vi "Subvi AO.vi"(2 "AO channel":refnum<k21>="Connector1/AO0", 8 "Ext trig enable":bool, 10 "Memory label":refnum<k21>="AO0 buffer") -> ()   [LabVIEW 2017]
uses:
  <vilib>/Platform/TimedLoop/XDataNode/timing_clust.ctl
  <vilib>/Platform/TimedLoop/XDataNode/nitl_modes.ctl
  <vilib>/Platform/TimedLoop/XDataNode/wakeup.ctl
  <vilib>/rvi/Emulation/niFpgaSctlEmulationGetInTimedLoop.vi
  <vilib>/rvi/Emulation/niFpgaEmulationReportErrorSimple.vi
  <vilib>/rvi/Emulation/niFpgaGetClockAttributes.vi
  <vilib>/rvi/Emulation/niFpgaCriticalErrorInLSC.vi
  Detector/GV line clock start.vi
  <vilib>/rvi/DataTransferAndStorage/Container/Common/niFpgaContainerExecOnDevCompGetState.vi
  <vilib>/rvi/Emulation/niFpgaEmulationIsFPGAContextNoSignature.vi
  <vilib>/rvi/DataTransferAndStorage/Container/Common/niFpgaContainerGetUniqueNameForEmu.vi
  <vilib>/rvi/Emulation/niFpgaProcessEmulError.vi
  <vilib>/rvi/errors/nirviReportUnexpectedCaseInternalError (U32).vi
  <vilib>/rvi/Memory/Memory_Emulation/niFpgaMemoryEmulationCacheClearOnFirstRun.vi
  <vilib>/rvi/Memory/Memory_Emulation/nirvimemoryEmulationManagerCache_MakeExclusive.vi
  <vilib>/rvi/Memory/Memory_Emulation/niFpgaMemoryEmulationValidateCache.vi
  <vilib>/rvi/Memory/Memory_Emulation/nirvimemoryEmulationManagerCache_InsertValue.vi
  <vilib>/Utility/error.llb/Clear Errors.vi
  <vilib>/rvi/Memory/Memory_Emulation/nirvimemoryEmulationManagerCache_ReleaseExclusive.vi
  <vilib>/rvi/Memory/Memory_Emulation/nirvimemoryEmulationManagerCache_GetValue.vi
  <vilib>/rvi/Memory/Memory_Emulation/nirvimemoryEmulationManagerCache_SetValue.vi
  <vilib>/rvi/Emulation/niFpgaSctlEmulationResourceMgr.vi
  <vilib>/rvi/eio/common/nirviEmuTemplateMethod_errors.vi
  <vilib>/Platform/TimedLoop/XDataNode/XDataNode.xnode
  <vilib>/rvi/DataTransferAndStorage/Container/XNode/niFpgaContainer.xnode
  <vilib>/rvi/Memory/Memory_Emulation/niFpgaMemoryEmulationRefIn.vi
  <vilib>/eio/EIONode/EIONode.xnode
  <vilib>/Platform/TimedLoop/XDataNode/XDNodeRunTimeDep.lvlib
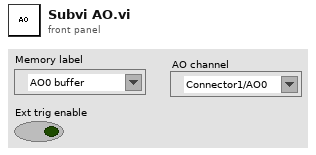
[diagram p1: front panel]
types:
  T1 = typedef "XDNodeRunTimeDep.lvlib/timing_clust.ctl" = cluster{"Expected End [f-1]":u64, "Actual End [f-1]":u64, "Finished Late? [f-1]":bool, "Expected End [i-1]":u64, "Actual End [i-1]":u64, "Finished Late? [i-1]":bool, "Expected Start [i]":u64, "Actual Start [i]":u64, "Expected Start [f]":u64, "Actual Start [f]":u64, "Source Name":string, "Structure Name":string, "Period":i64, "Deadline":i64, "Offset":i64, "Start":i64, "Priority":i32, "Timeout":i32, "Mode":T2, "Wakeup Reason":T3, "Error":errorcluster, "Source Type":string, "Secondary Source Type":string, "Global End Time":u64, "Global Start Time":u64, "Frame Duration":u64, "Iteration Duration":u64, "Assigned CPU":i32, "I/O Scan Engine Mode":u32}
  T2 = typedef "XDNodeRunTimeDep.lvlib/nitl_modes.ctl" = enum32{"No Change", "Process missed periods, maintain original phase", "Discard missed periods, maintain original phase", "Process missed periods, ignore original phase", "Discard missed periods, ignore original phase"}
  T3 = typedef "XDNodeRunTimeDep.lvlib/wakeup.ctl" = enum32{"Normal", "Aborted", "Asynchronous wakeup", "Timing source error", "Timed loop error", "Timeout"}
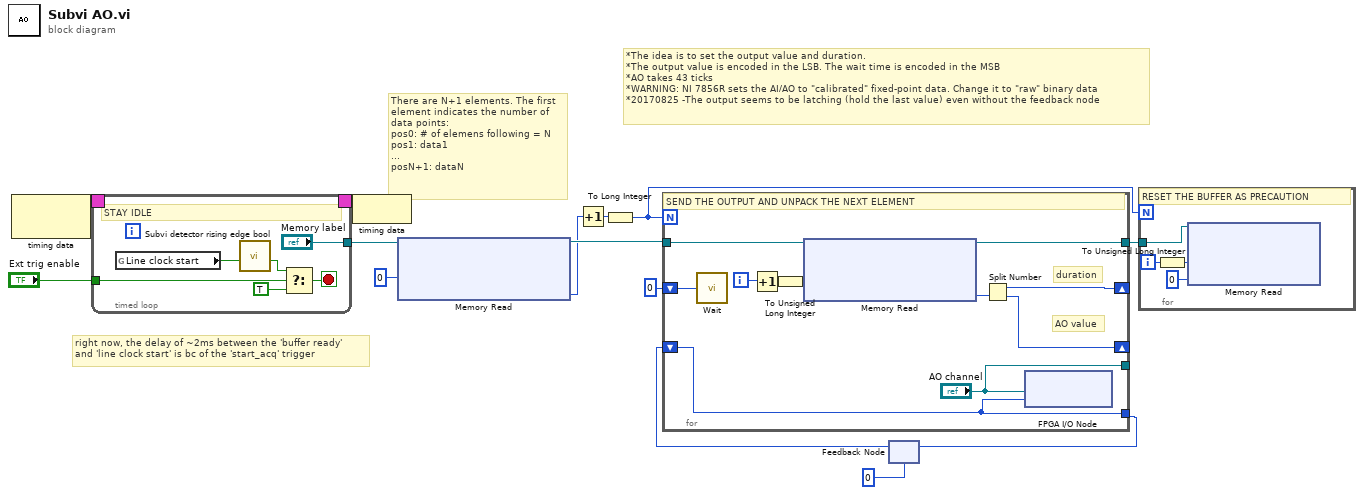
[diagram p0: block diagram]
diagram:
  # "right now, the delay of ~2ms between the 'buffer ready'\nand 'line clock start' is bc of the 'start_acq' trigger"
  # "There are N+1 elements. The first\nelement indicates the number of\ndata points:\npos0: # of elemens following = N\npos1: data1\n...\nposN+1: dataN"
  # "*The idea is to set the output value and duration.\n*The output value is encoded in the LSB. The wait time is encoded in the MSB\n*AO takes 43 ticks\n*WARNING: NI 7856R sets the AI/AO to \"calibrated\" fixed-point data. Change it to \"raw\" binary data\n*20170825 -The output seems to be latching (hold the last value) even without the feedback node"
  n1 = node-c288() -> (w3:T1)  [unwired: 1 in]
  n2 = timed-loop {
    tunnel: ["Memory label"] -> w4
    timing: w3 -> [_]
    timing-out: [_] -> w2
    tunnel: "Ext trig enable" -> [w18]
    stop <- w16 stop-if-true
    # "STAY IDLE"
    n3 = global read "GV line clock start.vi" "Line clock start"() -> (w20:bool)
    n4 = call "Subvi detector rising edge bool.vi"("Input"=w20) -> ("Output"=w17:bool)  [unwired: 10 in]
    n5 = Select(t=w17, s=w18, f=TRUE) -> (s? t:f=w16:bool)
  }
  n6 = node-c288(w2) -> ()
  n7 = xnode ("Memory Read")("Address"=u32 0, "Memory In"=w4) -> ("Data"=w10:u32, "Memory Out"=w12:refnum<k21>)
  n8 = Increment(x=w10) -> (x+1=w9:u32)
  n9 = To Long Integer(number=w9) -> (32bit integer=w8:i32)
  n10 = feedback #1(u16 0) -> (w7:u16)
  n11 = for {
    N: w8 -> [_]
    shift-right: [w32] -> _
    shift-left: u16 0 -> [w33]
    shift-right: [w30] -> _
    shift-left: w7 -> [w23]
    tunnel: ["AO channel"] -> _
    tunnel: [w29] -> w11
    tunnel: w12 -> [w27]
    tunnel: [w23] -> w5
    i -> [w26]
    # "duration"
    # "AO value"
    # "SEND THE OUTPUT AND UNPACK THE NEXT ELEMENT"
    n12 = call "Wait"("Count(Ticks)"=w33) -> ()  [unwired: 1 out]
    n13 = Increment(x=w26) -> (x+1=w25:i32)
    n14 = To Unsigned Long Integer(number=w25) -> (unsigned 32bit integer=w24:u32)
    n15 = xnode ("Memory Read")("Memory In"=w27, "Address"=w24) -> ("Memory Out"=w29:refnum<k21>, "Data"=w31:u32)
    n16 = Split Number(x=w31) -> (hi(x)=w32:u16, lo(x)=w30:u16)
    n17 = xnode "FPGA I/O Node"("I/O Item"=w23, "FPGA I/O In"="AO channel") -> ()  [unwired: 1 out]
  }
  n18 = feedback-in #1(w5) -> ()
  n19 = for {
    N: w8 -> [_]
    tunnel: w11 -> [w37]
    i -> [w35]
    # "RESET THE BUFFER AS PRECAUTION"
    n20 = To Unsigned Long Integer(number=w35) -> (unsigned 32bit integer=w34:u32)
    n21 = xnode ("Memory Read")("Address"=w34, "Data"=u32 0, "Memory In"=w37) -> ()  [unwired: 1 out]
  }
